vi "Calculate Limit Test Query.vi"(8 "error in":errorcluster, 10 "Calculation Channel":i32(ring) items=["Calc Channel 1", "Calc Channel 2", "Calc Channel 3", "Calc Channel 4"], 11 "Instrument Handle In":i32) -> (0 "error out":errorcluster, 1 "Measurement":i32, 2 "Source":i32, 3 "Instrument Handle Out":i32, 4 "Lower Limit":dbl, 5 "Count":u32, 6 "Upper Limit":dbl)   [LabVIEW 8.6, in "ZTScopeM.lvlib"]
doc: "Query the limit test configuration for the selected calculation channel."
uses:
  ZTScopeM.lvlib
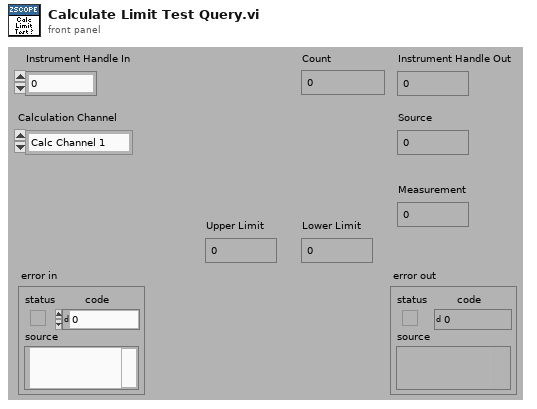
[diagram p1: front panel]
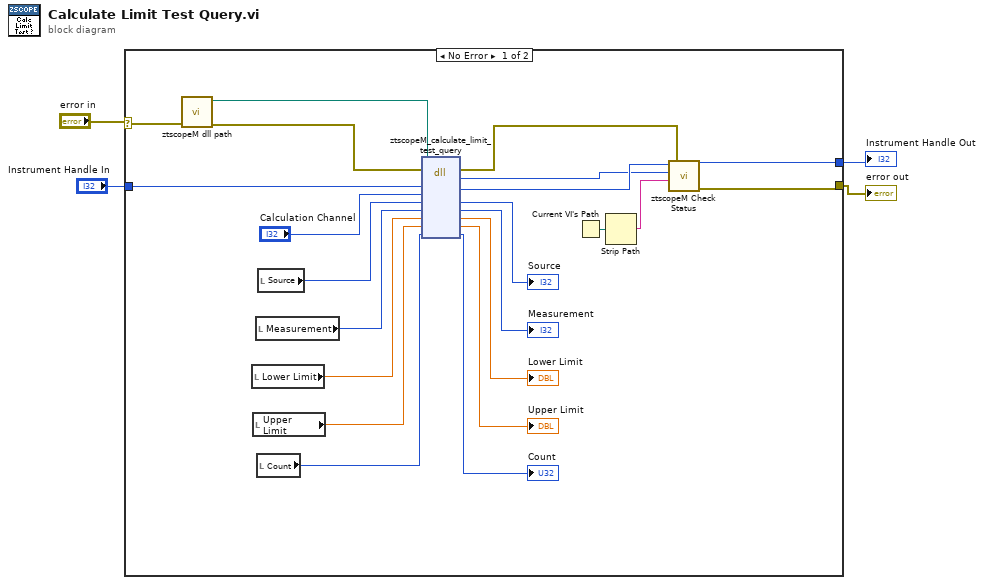
[diagram p0: block diagram]
diagram:
  n1 = case shown="No Error" "error in" {
    selector: "error in" -> [w8 w28]
    tunnel: [w12 w28] -> w2
    tunnel: "Instrument Handle In" -> [w26 w27]
    tunnel: [w11 w27] -> w1
    frame #0 {
      n2 = call "ztscopeM dll path.vi"("error in (no error)"=w8) -> ("error out"=w6:errorcluster, "<instrument>.dll path"=w7:path)  [unwired: 9 in]
      n3 = local read "Lower Limit"() -> (w20:dbl)
      n4 = local read "Upper Limit"() -> (w18:dbl)
      n5 = local read "Measurement"() -> (w22:i32)
      n6 = local read "Count"() -> (w9:u32)
      n7 = local read "Source"() -> (w24:i32)
      n8 = dll-call lib="C:/Program Files (x86)/National Instruments/LabVIEW 2013/instr.lib/ztscopem/ztscopeM.dll" fn="ztscopeM_calculate_limit_test_query"(path in=w7, error in=w6, "instrumentHandle"=w26, "calculationChannel"="Calculation Channel", "source"=w24, "Measurement"=w22, "lowerLimit"=w20, "upperLimit"=w18, "Count"=w9) -> (error out=w5:errorcluster, w13:i32, "instrumentHandle"=w14:i32, "source"=→"Source":i32, "Measurement"=→"Measurement":i32, "lowerLimit"=→"Lower Limit":dbl, "upperLimit"=→"Upper Limit":dbl, "Count"=→"Count":u32)  [unwired: 2 in, 1 out]
      n9 = Current VI's Path() -> (path=w16:path)
      n10 = Strip Path(path=w16) -> (name=w15:string)  [unwired: 1 out]
      n11 = call "ztscopeM Check Status.vi"("error in"=w5, "name of VI"=w15, "status (return code)"=w13, "instrument handle in"=w14) -> ("error out"=w12:errorcluster, "instrument handle out"=w11:i32)  [unwired: 2 in]
    }
    frame #1 {
    }
  }
  "Instrument Handle Out" <- w1
  "error out" <- w2
